vi "Create New Document.vi"(8 "error in (no error)":errorcluster, 10 "Document Type":T1, 11 "File Path":path) -> (0 "error out":errorcluster, 3 "Document out":refnum<class "Document API.lvclass">)   [LabVIEW 2017, in "Document API.lvlib" / "Document API.lvclass"]
doc: "Creates a new <b>Document out</b>, based on either the <b>Document Path</b> or <b>Document Type</b>. Use save to persist your changes.\n\nNotes:\n - The default file extensions for the <b>Document Type</b> are defined as follow: Word: *.docx, Excel: *.xlsx.\n - If the <b>Document Path</b> is empty (default) or is <Not A Path> or is a directory, the VI create a new document of the format specified by <b>Document Type</b>. Word will create a *.docx formated document. Excel will create a *.xlsx formatted document.\n - If the <b>Document Path</b> is a valid file path, the file extension is used to determine the file format to create. *.doc or *.docx will create a Word formated document. *.xls or *.xlsx will create an Excel formated document.\n - If the <b>Document Path</b> already contains a document with the same name then that file is overwritten without warning. Use Open Document to not overwrite an existing document."
uses:
  Document API.lvclass
  Document Type.ctl
  Document API.lvclass/Document API.ctl
  NPOI_Document/npoiDocument/npoiDocument.lvclass
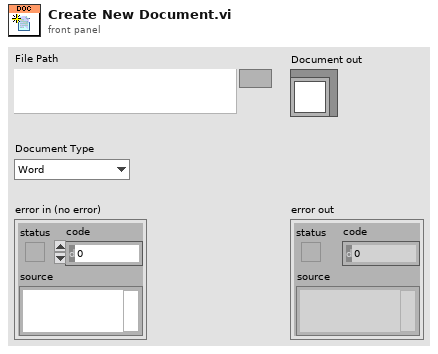
[diagram p1: front panel]
types:
  T1 = typedef "Document API.lvlib/Document API.lvclass/Document Type.ctl" = enum16{"Word", "Excel", "Undefined"}
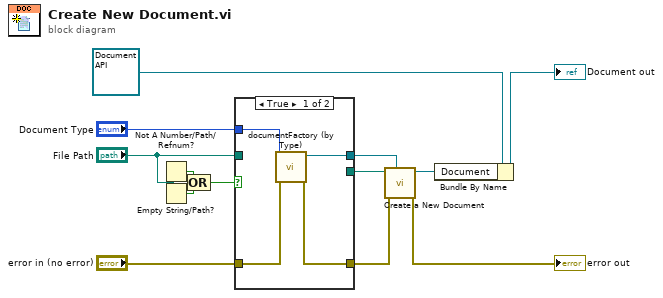
[diagram p0: block diagram]
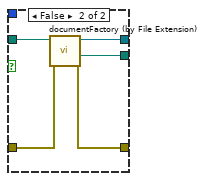
[diagram p2: hidden frame]
diagram:
  n1 = Not A Number/Path/Refnum?(number/path/refnum="File Path") -> (NaN/Path/Refnum?=w5:bool)
  n2 = Empty String/Path?(string/path="File Path") -> (empty?=w4:bool)
  n3 = Compound Arithmetic op=OR(w5, w4) -> (w2:bool)
  n4 = case shown="True" w2 {
    tunnel: "error in (no error)" -> [w17 w22]
    tunnel: [w16 w21] -> w10
    tunnel: [w15 w20] -> w7
    tunnel: [_ w19] -> w6
    tunnel: "File Path" -> [_ w18]
    tunnel: "Document Type" -> [w14 _]
    frame True {
      n5 = call "documentFactory (by Type).vi"("error in (no error)"=w17, "Document Type"=w14) -> ("error out"=w15:errorcluster, "npoiDocument out"=w16:refnum<class "npoiDocument.lvclass">)  [unwired: 8 in]
    }
    frame False {
      n6 = call "documentFactory (by File Extension).vi"("error in (no error)"=w22, "File Path"=w18) -> ("error out"=w20:errorcluster, "dup file"=w19:path, "npoiDocument out"=w21:refnum<class "npoiDocument.lvclass">)  [unwired: 7 in]
    }
  }
  n7 = call "Create a New Document.vi"("Document Type"=w10, "error in (no error)"=w7, "Document Path"=w6) -> ("error out"=→"error out":errorcluster, "Document out"=w9:refnum<class "npoiDocument.lvclass">)  [unwired: 7 in]
  n8 = Bundle By Name(cluster=refnum<class "Document API.lvclass"> refnum ("NPOI Document API in"), "Document"=w9) -> (→"Document out":refnum<class "Document API.lvclass">)
